vi "Message Handler.vi"(8 "error in (no error)":errorcluster, 11 "OOQMH in":refnum<class "OOQMH.lvclass">) -> (0 "error out":errorcluster, 3 "OOQMH out":refnum<class "OOQMH.lvclass">)   [LabVIEW 2024, in "OOQMH.lvlib" / "OOQMH.lvclass"]
uses:
  OOQMH.lvclass
  OOQMH.lvclass/OOQMH.ctl
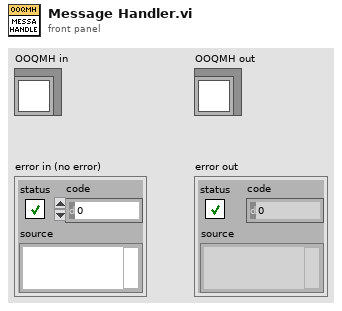
[diagram p1: front panel]
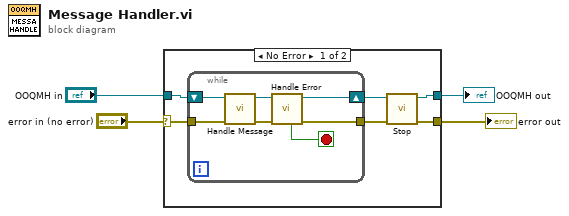
[diagram p0: block diagram]
diagram:
  n1 = case shown="No Error" "error in (no error)" {
    selector: "error in (no error)" -> [w9 w19]
    tunnel: [w5 w19] -> w3
    tunnel: [w6 w18] -> w1
    tunnel: "OOQMH in" -> [w10 w18]
    frame No Error {
      n2 = while {
        tunnel: [w15] -> w7
        shift-right: [w16] -> w8
        shift-left: w10 -> [w17]
        tunnel: w9 -> [w11]
        stop <- w14 stop-if-true
        n3 = call-dynamic "Handle Message.vi"("error in (no error)"=w11, "OOQMH in"=w17) -> ("error out"=w12:errorcluster, "OOQMH out"=w13:refnum<class "OOQMH.lvclass">)  [unwired: 8 in]
        n4 = call-dynamic "Handle Error.vi"("error in (no error)"=w12, "OOQMH in"=w13) -> ("error out"=w15:errorcluster, "OOQMH out"=w16:refnum<class "OOQMH.lvclass">, "stop?"=w14:bool)  [unwired: 7 in]
      }
      n5 = call-dynamic "Stop.vi"("error in (no error)"=w7, "OOQMH in"=w8) -> ("error out"=w5:errorcluster, "OOQMH out"=w6:refnum<class "OOQMH.lvclass">)  [unwired: 8 in]
    }
    frame Error {
    }
  }
  "error out" <- w3
  "OOQMH out" <- w1
